vi "Lex Comment-Text.vi"(8 "Error In":errorcluster) -> (0 "Error Out":errorcluster)   [LabVIEW 2018, in "Tests.lvlib" / "Lexer.lvlib"]
uses:
  Lexer.lvlib
  src/Toolkit/Low-Level/Tokens/Text/Text.lvclass
  src/Toolkit/Low-Level/Tokens/Comment/Comment.lvclass
  src/Toolkit/Low-Level/Support/Lex String.vi
  <vilib>/Utility/LVClass/Get LV Class Name.vi
  src/Toolkit/Low-Level/Tokens/Contentable/Contentable.lvclass
  <vilib>/addons/_JKI Toolkits/Caraya/classes/Test/Test.lvclass
  <vilib>/addons/_JKI Toolkits/Caraya/classes/Assert/Assert.lvclass
  Tests.lvlib
  src/Toolkit/Toolkit.lvlib
  src/Toolkit/Low-Level/Tokens/Abstract/Abstract.lvclass
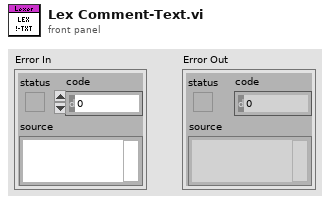
[diagram p1: front panel]
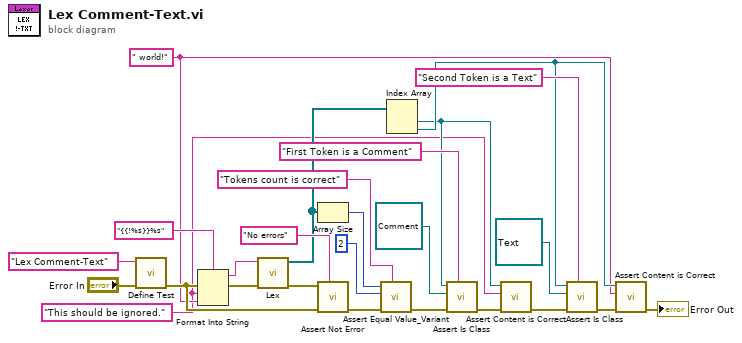
[diagram p0: block diagram]
diagram:
  w3 = " world!"
  w1 = "This should be ignored." ("format string")
  n1 = call <vilib>:"Define Test.vi"("error in (no error)"="Error In", "Label (VI Title)"="Lex Comment-Text") -> ("error out"=w13:errorcluster)  [unwired: 9 in]
  n2 = Format Into String(format string="{{!%s}}%s", error in=w13, w1, w3) -> (resulting string=w2:string, error out=w5:errorcluster)  [unwired: 1 in]
  n3 = call-poly "Lex.vi"("Error In"=w5, "Input"=w2) -> ("Error Out"=w24:errorcluster, "Tokens"=w18:refnum<class "Abstract.lvclass">[])  [unwired: 8 in]
  n4 = Array Size(array=w18) -> (size(s)=w20:i32)
  n5 = call <vilib>:"Assert Not Error.vi"("Label"="No errors", "error in (no error)"=w13, "Not Error?"=w24) -> ("error out"=w22:errorcluster)  [unwired: 8 in]
  n6 = call <vilib>:"Assert Equal Value_Variant.vi"("Label"="Tokens count is correct", "error in (no error)"=w22, "Y"=2 ("size(s)"), "X"=w20) -> ("error out"=w11:errorcluster)  [unwired: 7 in]
  n7 = Index Array(array=w18) -> (element #1=w6:refnum<class "Abstract.lvclass">, element #2=w12:refnum<class "Abstract.lvclass">)  [unwired: 2 in]
  n8 = call "Assert Is Class.vi"("Label"="First Token is a Comment", "Error In"=w11, "Expected"=refnum<class "Comment.lvclass"> refnum ("Toolkit.lvlib:Tokens.lvlib:Comment.lvclass"), "Actual"=w6) -> ("Error Out"=w8:errorcluster)  [unwired: 7 in]
  n9 = call "Assert Content is Correct.vi"("Error In"=w8, "Expected"=w1, "Token"=w6) -> ("Error Out"=w7:errorcluster)  [unwired: 8 in]
  n10 = call "Assert Is Class.vi"("Label"="Second Token is a Text", "Error In"=w7, "Expected"=refnum<class "Text.lvclass"> refnum ("Mustache.lvlib:Tokens.lvlib:Text.lvclass"), "Actual"=w12) -> ("Error Out"=w16:errorcluster)  [unwired: 7 in]
  n11 = call "Assert Content is Correct.vi"("Error In"=w16, "Expected"=w3, "Token"=w12) -> ("Error Out"=→"Error Out":errorcluster)  [unwired: 8 in]
